vi "Database.vi"(3 "error in (no error)":errorcluster, 5 "table":string) -> (0 "error out":errorcluster, 1 "data":string[][](array[string]), 2 "recordset reference out":T1)   [LabVIEW 2019]
uses:
  <vilib>/addons/database/Recordset.llb/Rec ObjectReference.ctl
  <vilib>/addons/database/Connection.llb/DB Tools Open Connec (String).vi
  <vilib>/addons/database/Connection.llb/Conn Execute.vi
  <vilib>/addons/database/Recordset.llb/Rec Fetch Recordset Data (R).vi
  <vilib>/addons/database/NI_Database_API.lvlib
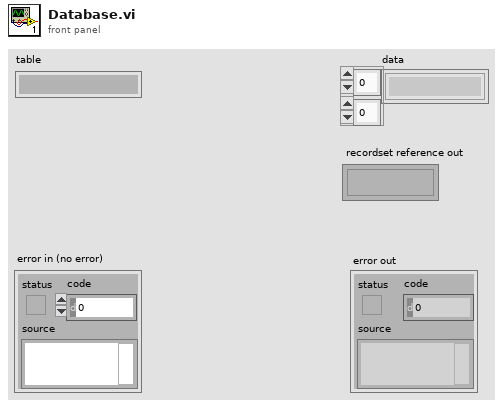
[diagram p1: front panel]
types:
  T1 = typedef "NI_Database_API.lvlib/Rec ObjectReference.ctl" = refnum<k1>
  T2 = typedef "NI_Database_API.lvlib/Conn ObjectReference.ctl" = refnum<k1>
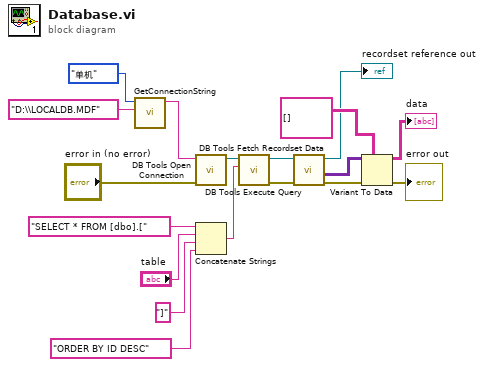
[diagram p0: block diagram]
diagram:
  n1 = call "GetConnectionString.vi"("Database Name"="D:\\LOCALDB.MDF", "连接模式"=enum16{"单机", "联网"}."单机") -> ("连接字符串"=w4:string)  [unwired: 4 in, 1 out]
  n2 = call-poly <vilib>:"DB Tools Open Connection.vi"("error in (no error)"="error in (no error)", "connection information"=w4) -> ("connection reference"=w11:T2)  [unwired: 6 in, 1 out]
  n3 = Concatenate Strings("SELECT * FROM [dbo].[", "table", "]", "ORDER BY ID DESC" ("字符串")) -> (w5:string)
  n4 = call-poly <vilib>:"DB Tools Execute Query.vi"("SQL query"=w5, "connection reference"=w11) -> ("error out"=w17:errorcluster, "recordset reference"=w16:T1)  [unwired: 6 in]
  n5 = call-poly <vilib>:"DB Tools Fetch Recordset Data.vi"("error in (no error)"=w17, "recordset reference"=w16) -> ("error out"=w15:errorcluster, "recordset data"=w14:variant[][], "recordset reference out"=→"recordset reference out":T1)  [unwired: 3 in]
  n6 = Variant To Data(error in=w15, type=string[][] [], Variant=w14) -> (data=→"data":string[][], error out=→"error out":errorcluster)
